vi "Address Space Size.vi"(2 "WaveformAddressSpace":refnum<class "WaveformAddressSpace.lvclass">) -> (6 "size":u32)   [LabVIEW 2017, in "WaveformAddressSpace.lvclass"]
uses:
  WaveformAddressSpace.lvclass
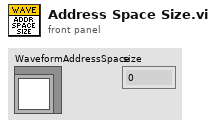
[diagram p1: front panel]
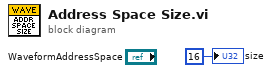
[diagram p0: block diagram]
diagram:
  "size" <- u32 16 ("size")
